vi "Deserialize.vi"(8 "error in (no error)":errorcluster, 10 "Serialized PE Spec":string, 11 "RandomNumberLogger Controller in":refnum<class "RandomNumberLogger Controller.lvclass">) -> (0 "error out":errorcluster, 3 "RandomNumberLogger Controller out":refnum<class "RandomNumberLogger Controller.lvclass">)   [LabVIEW 2020, in "RandomNumberLogger.lvlib" / "RandomNumberLogger Controller.lvclass"]
doc: "<b>Deserailize</b>\nThis VI loads the configuration that has been deserialized into the plugin controller object."
uses:
  RandomNumberLogger Controller.lvclass
  RandomNumberLogger Controller.lvclass/RandomNumberLogger Controller.ctl
  PE/Get Configuration Version.vi
  PE/Mutate Configuration to Current.vi
  PE/Default Configuration Parameters.vi
  <vilib>/ADAS Record/Utilities/Config/Data Converter/Populate Container from JSON.vi
  PE/RandomNumberLogger.lvclass
panel:
  # "#via_ignore"
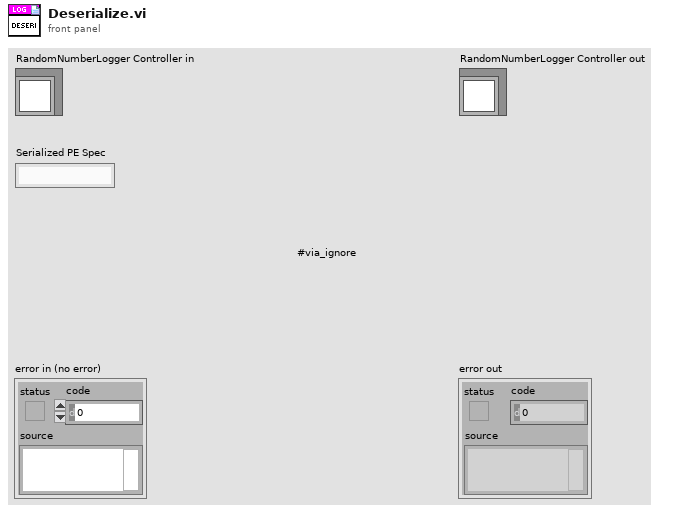
[diagram p1: front panel]
types:
  T1 = typedef "RandomNumberLogger.lvlib/RandomNumberLogger.lvclass/Configuration.ctl" = cluster{"Parameter1":string}
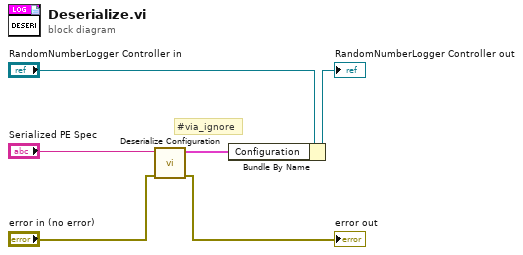
[diagram p0: block diagram]
diagram:
  # "#via_ignore"
  n1 = call "Deserialize Configuration.vi"("error in (no error)"="error in (no error)", "Serialized Configuration"="Serialized PE Spec") -> ("error out"=→"error out":errorcluster, "Configuration"=w3:T1)  [unwired: 8 in]
  n2 = Bundle By Name(cluster="RandomNumberLogger Controller in", "Configuration"=w3) -> (→"RandomNumberLogger Controller out":refnum<class "RandomNumberLogger Controller.lvclass">)
